vi "LDPC_matlab_input.vi"() -> (4 "Value output":dbl, 10 "Change output":bool)   [LabVIEW 2018]
panel:
  in  "Value":string caption="\"y\" value"
  in  "Change":bool
  # "LDPC TIMINGS"
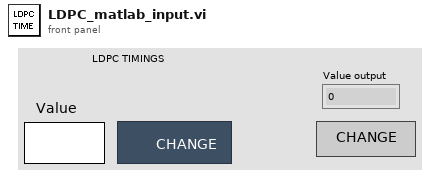
[diagram p1: front panel]
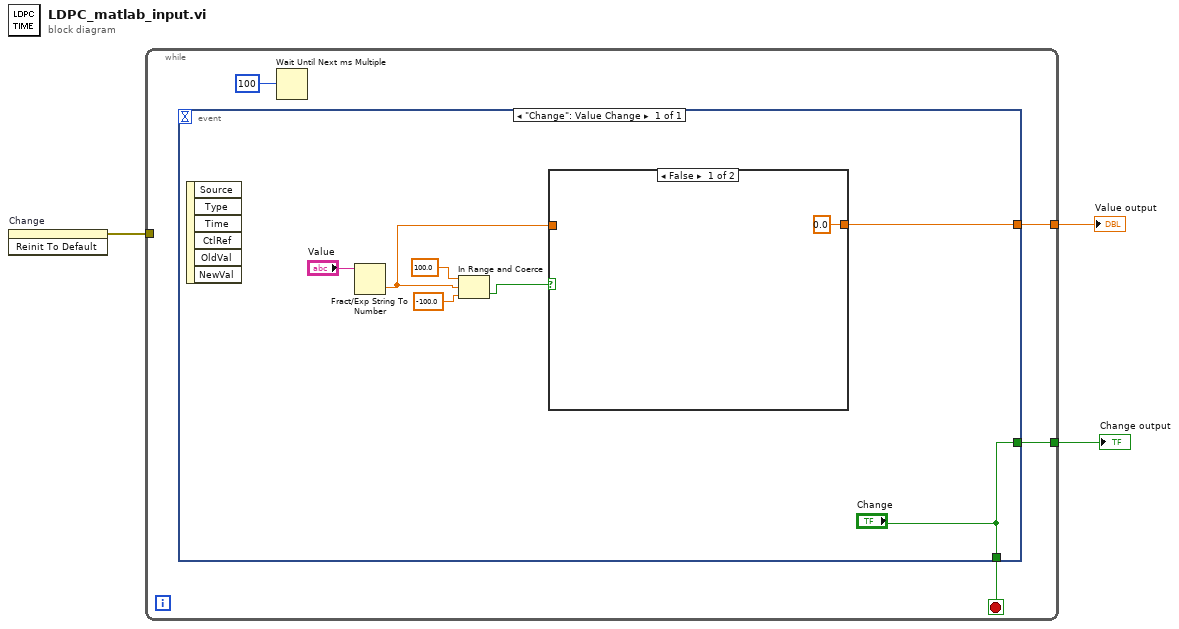
[diagram p0: block diagram]
diagram:
  n1 = invoke on="Change" class="Bool" method="Reinit To Default"() -> (error out=w3:errorcluster)  [unwired: 3 in, 2 out]
  n2 = while {
    tunnel: w3 -> [_]
    tunnel: [w6] -> w2
    tunnel: [w4] -> w1
    stop <- w5 stop-if-true
    n3 = event shown="[0] \"Change\": Value Change" {
      selector: _ -> [_]
      dyn-events: _ -> [_]
      timeout: _ -> [_]
      tunnel: [w8] -> w6
      tunnel: ["Change"] -> w5
      tunnel: ["Change"] -> w4
      event "Change": Value Change {
        n4 = event-data() -> ()  [unwired: 1 in, 6 out]
        n5 = Fract/Exp String To Number(string="Value") -> (number=w9:dbl)  [unwired: 3 in, 1 out]
        n6 = In Range and Coerce(upper limit=100.0, x=w9, lower limit=-100.0) -> (In Range?=w10:bool)  [unwired: 1 out]
        n7 = case shown="False" w10 {
          tunnel: [0.0 w16] -> w8
          tunnel: w9 -> [_ w16]
          frame False {
          }
          frame True {
          }
        }
      }
    }
    n8 = Wait Until Next ms Multiple(millisecond multiple=100) -> ()  [unwired: 1 out]
  }
  "Change output" <- w1
  "Value output" <- w2
